vi "Ramp_Trajectory.vi"(7 "Initial Time (s)":dbl, 8 "Period (s)":dbl, 9 "Ramp Duration (s)":dbl, 10 "Final Position (deg)":dbl, 11 "Initial Position (deg)":dbl) -> (3 "Profile":cluster{"time (s)":dbl, "setpoint":dbl}[](array[cluster]) {"setpoint" format="%.2f"; "time (s)" format="%.3f"})   [LabVIEW 2019]
uses:
  <vilib>/Analysis/1siggen.llb/Ramp Pattern by Samples.vi
  <vilib>/Analysis/NI_AALBase.lvlib
panel:
  out "XY Graph":cluster{"X":dbl, "Y":dbl}[](graph)
  out "Waveform Graph":waveform(dbl)(graph)
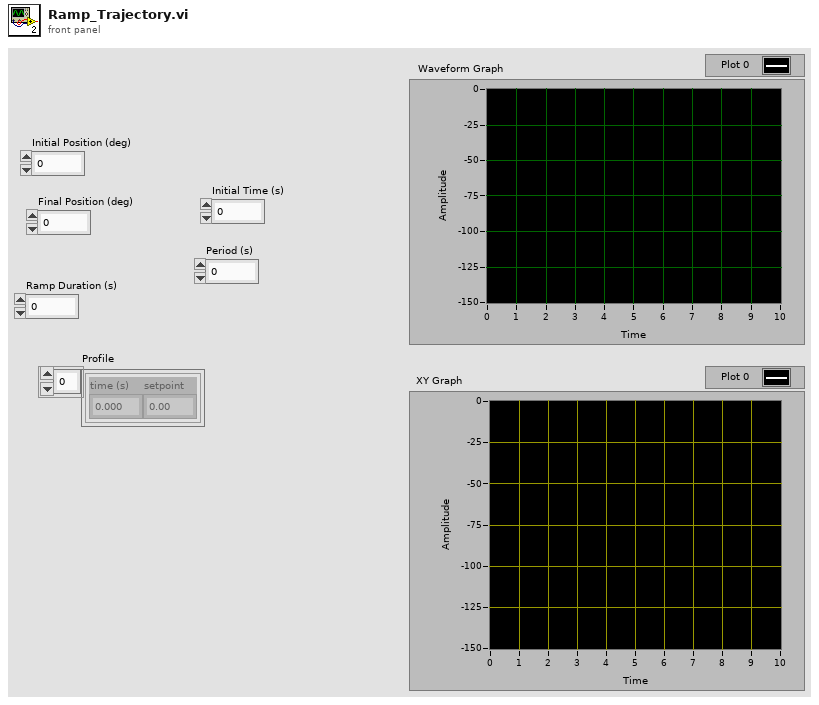
[diagram p1: front panel]
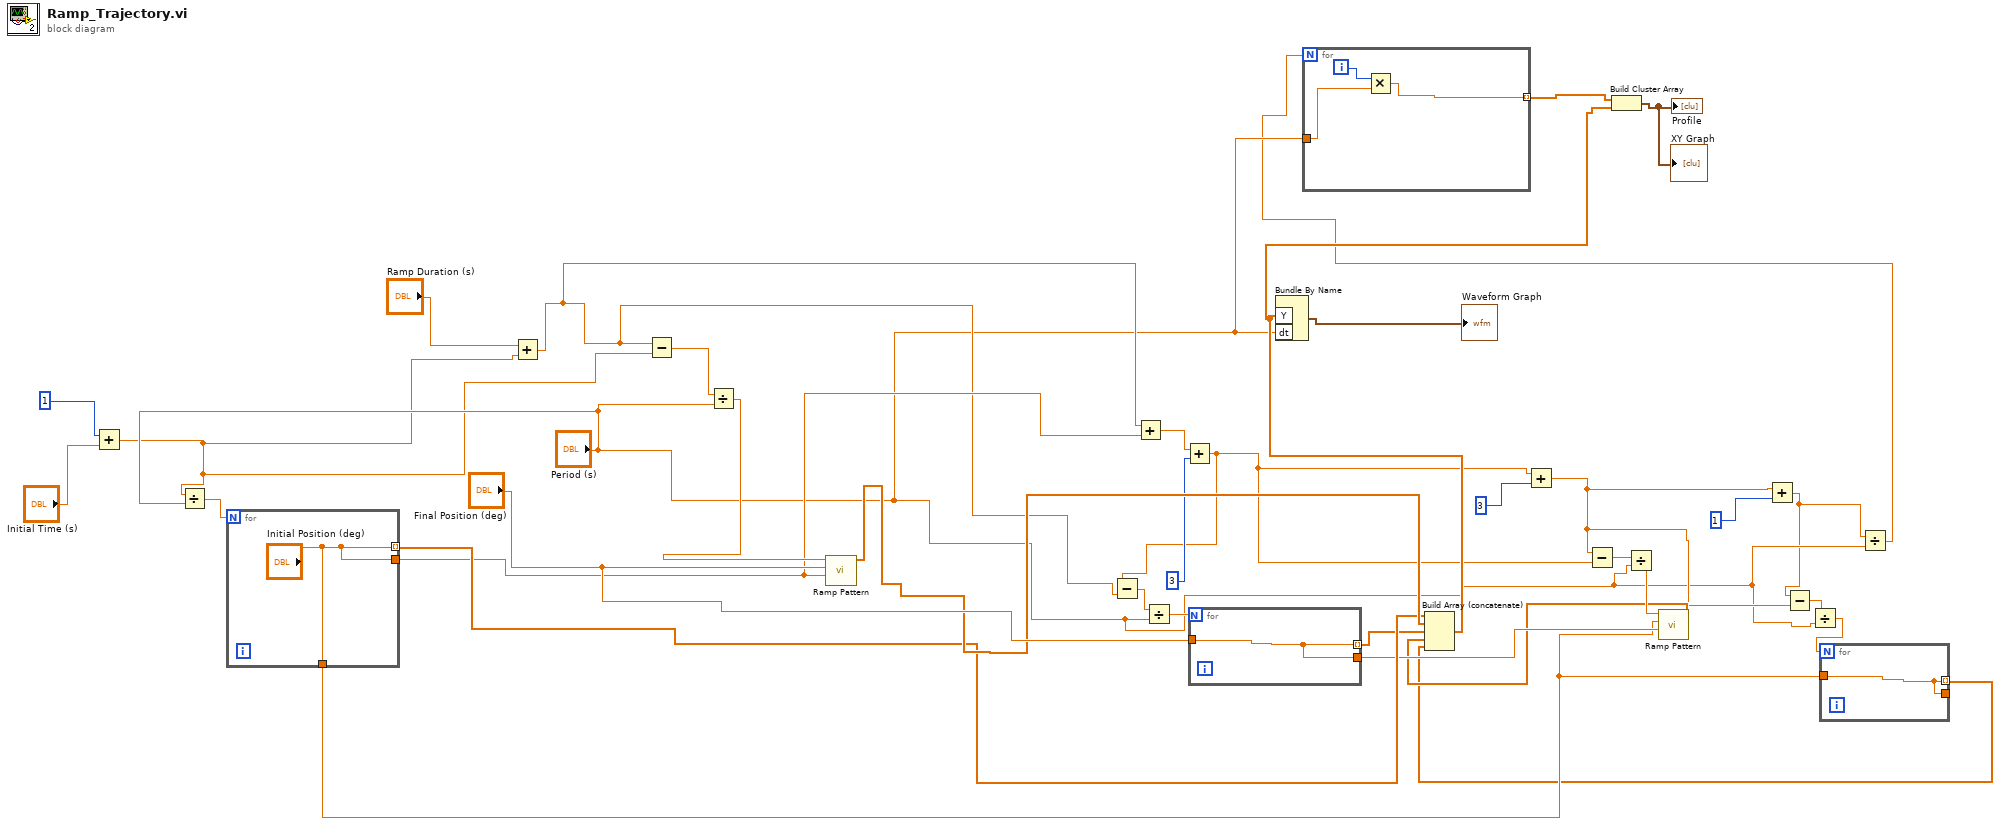
[diagram p0: block diagram]
diagram:
  n1 = Add(x=1, y="Initial Time (s)") -> (x+y=w3:dbl)
  n2 = Divide(x=w3, y="Period (s)") -> (x/y=w34:dbl)
  n3 = for {
    N: w34 -> [_]
    tunnel: ["Initial Position (deg)"] -> w29 mode=indexing
    tunnel: ["Initial Position (deg)"] -> w21
    tunnel: ["Initial Position (deg)"] -> w24
  }
  n4 = Add(x="Ramp Duration (s)", y=w3) -> (x+y=w17:dbl)
  n5 = Subtract(x=w17, y=w3) -> (x-y=w36:dbl)
  n6 = Divide(x=w36, y="Period (s)") -> (x/y=w35:dbl)
  n7 = call-poly <vilib>:"Ramp Pattern.vi"("start"=w21, "end"="Final Position (deg)", "samples"=w35) -> ("Ramp Pattern"=w30:dbl[])  [unwired: 7 in, 1 out]
  n8 = Add(x=w17, y=w21) -> (x+y=w19:dbl)
  n9 = Add(x=w19, y=3) -> (x+y=w1:dbl)
  n10 = Subtract(x=w1, y=w17) -> (x-y=w32:dbl)
  n11 = Divide(x=w32, y="Period (s)") -> (x/y=w31:dbl)
  n12 = for {
    N: w31 -> [_]
    tunnel: [w38] -> w2 mode=indexing
    tunnel: [w38] -> w28
    tunnel: "Final Position (deg)" -> [w38]
  }
  n13 = Add(x=w1, y=3) -> (x+y=w15:dbl)
  n14 = Subtract(x=w15, y=w1) -> (x-y=w27:dbl)
  n15 = Divide(x=w27, y="Period (s)") -> (x/y=w26:dbl)
  n16 = call-poly <vilib>:"Ramp Pattern.vi"("start"=w28, "end"=w24, "samples"=w26) -> ("Ramp Pattern"=w23:dbl[])  [unwired: 7 in, 1 out]
  n17 = Add(x=w15, y=1) -> (x+y=w7:dbl)
  n18 = Subtract(x=w7, y=w15) -> (x-y=w25:dbl)
  n19 = Divide(x=w25, y="Period (s)") -> (x/y=w9:dbl)
  n20 = for {
    N: w9 -> [_]
    tunnel: [w39] -> w22 mode=indexing
    tunnel: [w39] -> _
    tunnel: w24 -> [w39]
  }
  n21 = Build Array (concatenate)(w29, w30, w2, w23, w22) -> (w10:dbl[])
  n22 = Bundle By Name("Y"=w10, "dt"="Period (s)") -> (→"Waveform Graph":waveform(dbl))  [unwired: 1 in]
  n23 = Divide(x=w7, y="Period (s)") -> (x/y=w6:dbl)
  n24 = for {
    N: w6 -> [_]
    tunnel: "Period (s)" -> [w41]
    tunnel: [w40] -> w11 mode=indexing
    i -> [w42]
    n25 = Multiply(x=w42, y=w41) -> (x*y=w40:dbl)
  }
  n26 = Build Cluster Array(w11, w10) -> (→"Profile" →"XY Graph":cluster{dbl, "Initial Position (deg)":dbl}[])
